vi "Apply filter data.vi"(8 "Weekday filter":T1, 9 "Quarter Filter":T2 {"month ring" items=["Jan", "Feb", "Mar", "Apr", "May", "Jun", "Jul", "Ago", "Set", "Oct", "Nov", "Dec"]}, 10 "data":dbl[][](array[numeric]), 11 "dates in":string[](array[string])) -> (2 "data out":dbl[][](array[numeric]), 3 "dates out":string[](array[string]))   [LabVIEW 2018]
panel:
  out "Array":i32[](array[numeric])
  out "appended array 2":string[](array[string])
  out "x .or. y?":bool
  out "Intensity Graph":dbl[][](graph)
  out "appended array":string[](array[string])
  out "logical OR 2":bool
  out "logical OR":bool
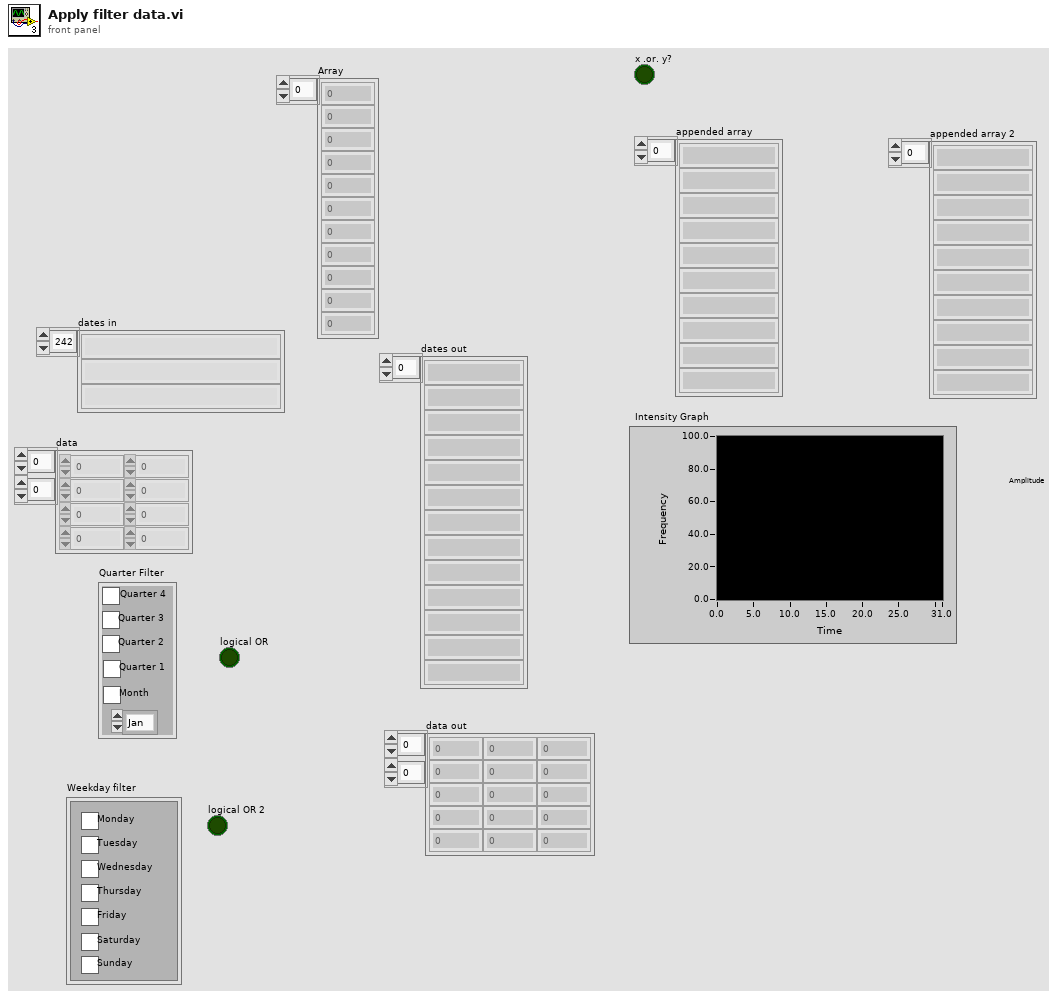
[diagram p1: front panel]
types:
  T1 = cluster{"Monday":bool, "Tuesday":bool, "Wednesday":bool, "Thursday":bool, "Friday":bool, "Saturday":bool, "Sunday":bool}
  T2 = cluster{"Q1 3":bool, "Q2 2":bool, "Q3 2":bool, "Q4 2":bool, "Q1 4":bool, "month ring":u16}
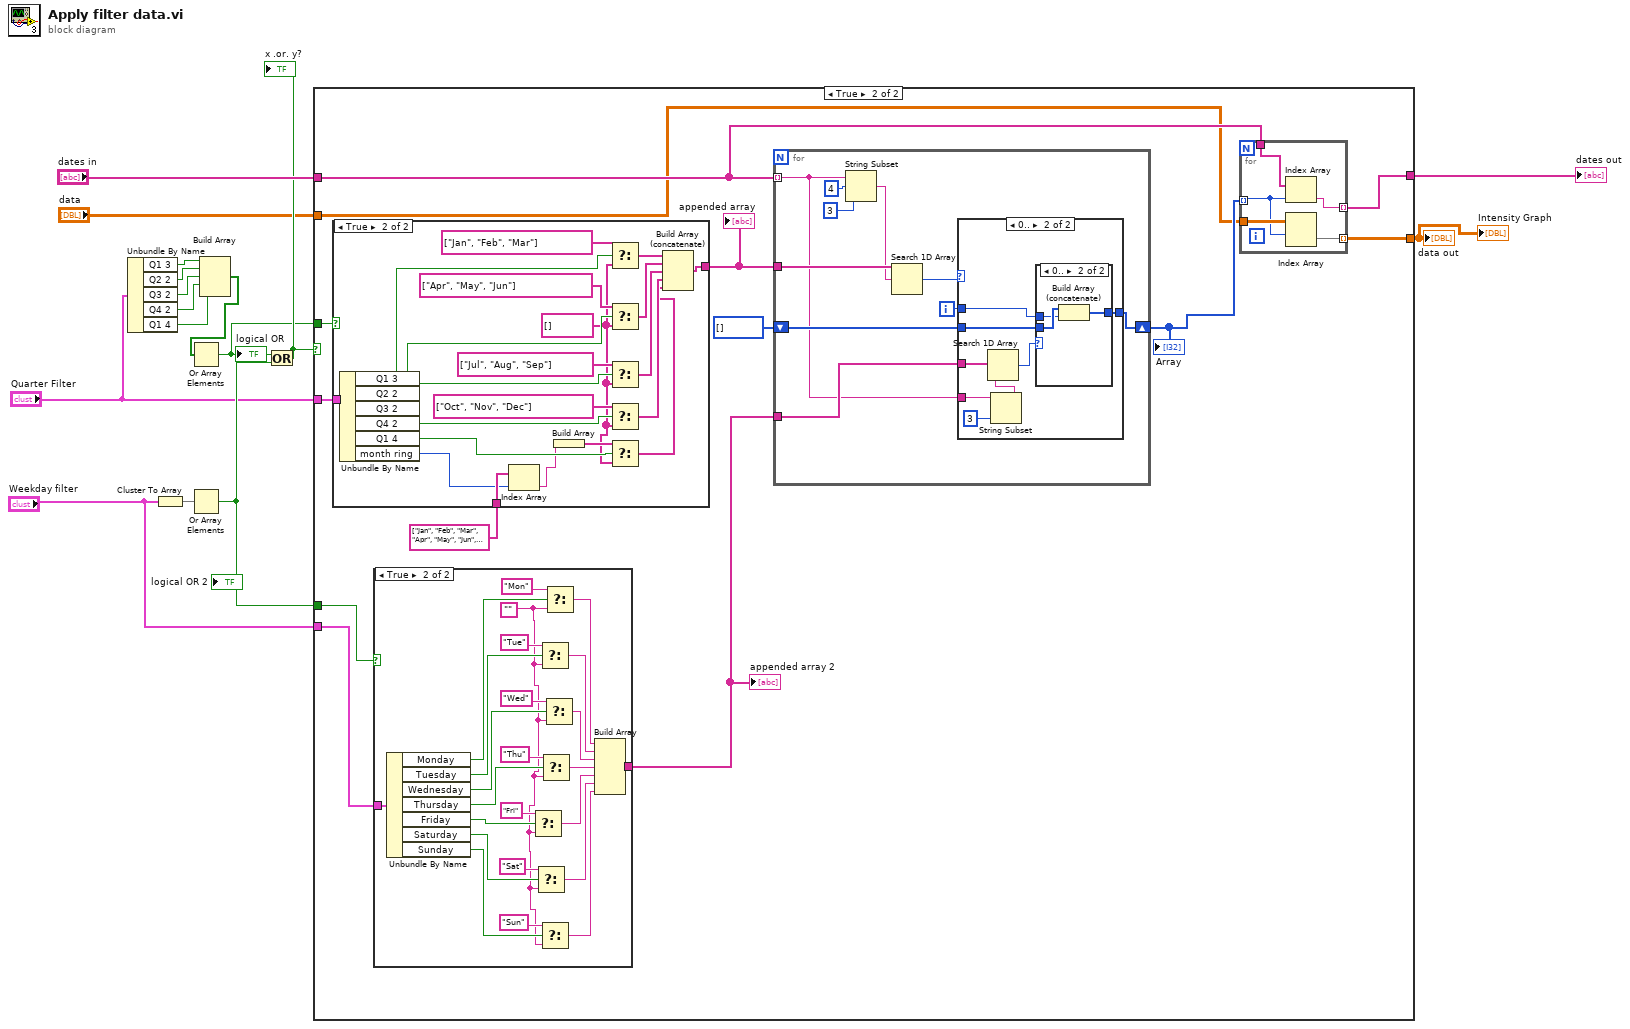
[diagram p0: block diagram]
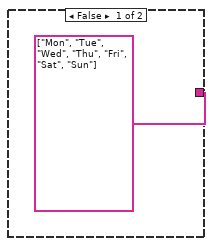
[diagram p4: hidden frame]
diagram:
  n1 = Unbundle By Name("Quarter Filter") -> ("Q1 3"=w6:bool, "Q2 2"=w5:bool, "Q3 2"=w4:bool, "Q4 2"=w3:bool, "Q1 4"=w2:bool)
  n2 = Cluster To Array(cluster="Weekday filter") -> (array=w15:bool[])
  n3 = Or Array Elements(Boolean array=w15) -> (logical OR=w10:bool)
  "logical OR 2" <- w10
  n4 = Build Array(w6, w5, w4, w3, w2) -> (w1:bool[])
  n5 = Or Array Elements(Boolean array=w1) -> (logical OR=w9:bool)
  "logical OR" <- w9
  n6 = Or(x=w9, y=w10) -> (x .or. y?=w14:bool)
  "x .or. y?" <- w14
  n7 = case shown="True" w14 {
    tunnel: "Quarter Filter" -> [_ w31]
    tunnel: "dates in" -> [w18 w25]
    tunnel: "Weekday filter" -> [_ w28]
    tunnel: [w18 w24] -> w12
    tunnel: "data" -> [w17 w23]
    tunnel: [w17 w22] -> w8
    tunnel: w10 -> [_ w21]
    tunnel: w9 -> [_ w20]
    frame False {
    }
    frame True {
      n8 = case shown="True" w20 {
        tunnel: w31 -> [_ w42]
        tunnel: [w32 w41] -> w30
        tunnel: string[] ["Jan", "Feb", "Mar", "Apr", "May", "Jun", "Jul", "Aug", "Sep", "Oct", "Nov", "Dec"] ("appended array") -> [w32 w38]
        frame False {
        }
        frame True {
          w34 = string[] []
          n9 = Unbundle By Name(w42) -> ("Q1 3"=w43:bool, "Q2 2"=w45:bool, "Q3 2"=w46:bool, "Q4 2"=w47:bool, "Q1 4"=w39:bool, "month ring"=w37:u16)
          n10 = Index Array(array=w38, index=w37) -> (element=w36:string)
          n11 = Build Array(w36) -> (w35:string[])
          n12 = Select(t=string[] ["Jan", "Feb", "Mar"], s=w43, f=w34) -> (s? t:f=w51:string[])
          n13 = Select(t=string[] ["Apr", "May", "Jun"], s=w45, f=w34) -> (s? t:f=w52:string[])
          n14 = Select(t=string[] ["Jul", "Aug", "Sep"], s=w46, f=w34) -> (s? t:f=w53:string[])
          n15 = Select(t=string[] ["Oct", "Nov", "Dec"], s=w47, f=w34) -> (s? t:f=w40:string[])
          n16 = Select(t=w35, s=w39, f=w34) -> (s? t:f=w33:string[])
          n17 = Build Array (concatenate)(w51, w52, w53, w40, w33) -> (w41:string[])
        }
      }
      "appended array" <- w30
      n18 = case shown="True" w21 {
        tunnel: w28 -> [_ w78]
        tunnel: [string[] ["Mon", "Tue", "Wed", "Thu", "Fri", "Sat", "Sun"] ("appended array 2") w77] -> w27
        frame False {
        }
        frame True {
          w55 = ""
          n19 = Unbundle By Name(w78) -> ("Monday"=w76:bool, "Tuesday"=w68:bool, "Wednesday"=w67:bool, "Thursday"=w66:bool, "Friday"=w65:bool, "Saturday"=w64:bool, "Sunday"=w63:bool)
          n20 = Select(t="Fri" ("String"), s=w65, f=w55) -> (s? t:f=w58:string)
          n21 = Select(t="Sat" ("String"), s=w64, f=w55) -> (s? t:f=w57:string)
          n22 = Select(t="Tue" ("String"), s=w68, f=w55) -> (s? t:f=w61:string)
          n23 = Select(t="Sun" ("String"), s=w63, f=w55) -> (s? t:f=w56:string)
          n24 = Select(t="Thu" ("String"), s=w66, f=w55) -> (s? t:f=w59:string)
          n25 = Select(t="Wed" ("String"), s=w67, f=w55) -> (s? t:f=w60:string)
          n26 = Select(t="Mon" ("String"), s=w76, f=w55) -> (s? t:f=w62:string)
          n27 = Build Array(w62, w61, w60, w59, w58, w57, w56) -> (w77:string[])
        }
      }
      "appended array 2" <- w27
      n28 = for {
        tunnel: w25 -> [w84] mode=indexing
        tunnel: w30 -> [w91]
        shift-right: [w87] -> w26
        shift-left: i32[] [] -> [w86]
        tunnel: w27 -> [w85]
        i -> [w88]
        n29 = String Subset(string=w84, offset (0)=4, length (rest)=3 ("length (rest)")) -> (substring=w90:string)
        n30 = Search 1D Array(1D array=w91, element=w90) -> (index of element=w89:i32)  [unwired: 1 in]
        n31 = case shown="0.." w89 {
          tunnel: w88 -> [_ w100]
          tunnel: [w94 w102] -> w87
          tunnel: w86 -> [w94 w101]
          tunnel: w85 -> [_ w99]
          tunnel: w84 -> [_ w97]
          frame -1, Default {
          }
          frame 0.. {
            n32 = String Subset(string=w97, length (rest)=3 ("length (rest)")) -> (substring=w95:string)  [unwired: 1 in]
            n33 = Search 1D Array(1D array=w99, element=w95) -> (index of element=w96:i32)  [unwired: 1 in]
            n34 = case shown="0.." w96 {
              tunnel: [w103 w106] -> w102
              tunnel: w101 -> [w103 w105]
              tunnel: w100 -> [_ w104]
              frame -1, Default {
              }
              frame 0.. {
                n35 = Build Array (concatenate)(w105, w104) -> (w106:i32[])
              }
            }
          }
        }
      }
      "Array" <- w26
      n36 = for {
        tunnel: w26 -> [w80] mode=indexing
        tunnel: w25 -> [w83]
        tunnel: [w82] -> w24 mode=indexing
        tunnel: w23 -> [w81]
        tunnel: [w79] -> w22 mode=indexing
        n37 = Index Array(array=w83, index=w80) -> (element=w82:string)
        n38 = Index Array(array=w81, index (row)=w80) -> (element=w79:dbl[])  [unwired: 1 in]
      }
    }
  }
  "dates out" <- w12
  "data out" <- w8
  "Intensity Graph" <- w8
